vi "Vision Research Phantom Series PhCon PhGetVersion.vi"(0 "CN in":u32=1, 2 "VerSel":T1 items=["GV_CAMERA"=1, "GV_FIRMWARE"=2, "GV_FPGA"=3, "GV_PHCON"=4, "GV_CFA"=5, "GV_KERNEL"=6, "GV_MAGAZINE"=7], 5 "Error In (no error)":errorcluster) -> (14 "CN out":u32=1, 16 "pVersion":u32, 19 "Error Out":errorcluster)   [LabVIEW 2013, in "VRI.lvlib"]
doc: "PhCon.dll\n\nPhGetVersion\nHRESULT PhGetVersion(UINT CN, UINT VerSel UINT*pVersion);\n\nParameters Description\nCN (in) Camera number.\nVerSel (in) Code to select the wanted version.\npVersion (out) The version requested.\nReturn HRESULT (0=Ok)\nComments Get the versions of the camera hardware, firmware, dll, \n FPGAs or sensor CFA. Set the VerSel parameter to one \n of the below values:\n GV_CAMERA–get the camera hardware version\n GV_FIRMWARE-get the firmware version\n GV_FPGA-get the FPGAs version\n GV_PHCON-get the dll version\n GV_CFA-get the sensor CFA\n\n\nWritten by:\nBLOOMY CONTROLS, INC\nWINDSOR, CT 06095, USA\n860-298-9925\nwww.bloomy.com\nV1.0.0\nMay, 2004"
uses:
  VRI.lvlib
  _Type Defs/PhCon VerSel.ctl
  Phantom DLLs/PhCon.Dll
panel:
  # "For instructions on the use of this VI, press Ctrl+H to display the help window and move the mouse over the icon, controls, and indicators"
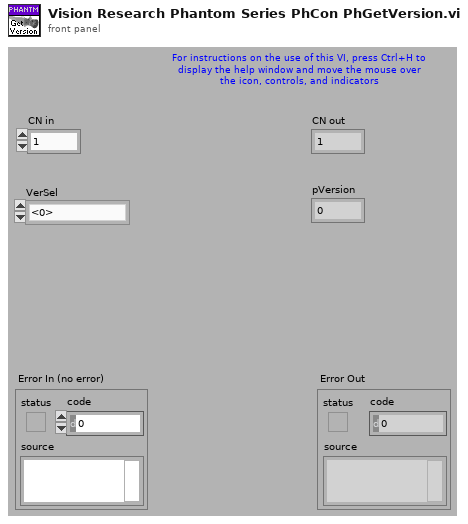
[diagram p1: front panel]
types:
  T1 = typedef "VRI.lvlib/PhCon VerSel.ctl" = u16
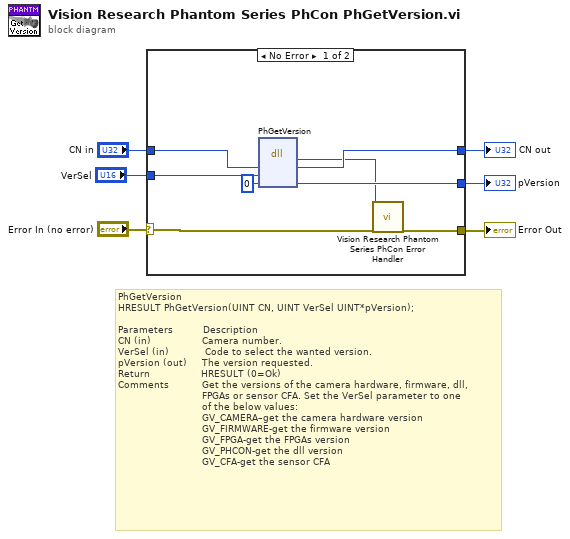
[diagram p0: block diagram]
diagram:
  # "PhGetVersion\nHRESULT PhGetVersion(UINT CN, UINT VerSel UINT*pVersion);\n\nParameters          Description\nCN (in)                 Camera number.\nVerSel (in)            Code to select the wanted version.\npVersion (out)     The version requested.\nReturn                 HRESULT (0=Ok)\nComments           Get the versions of the camera hardware, firmware, dll, \n                            FPGAs or sensor CFA. Set the VerSel parameter to one \n                            of the below values:\n                            GV_CAMERA–get the camera hardware version\n                            GV_FIRMWARE-get the firmware version\n                            GV_FPGA-get the FPGAs version\n                            GV_PHCON-get the dll version\n                            GV_CFA-get the sensor CFA"
  n1 = case shown="No Error" "Error In (no error)" {
    selector: "Error In (no error)" -> [w14 w16]
    tunnel: [w13 w16] -> w5
    tunnel: "CN in" -> [w12 w15]
    tunnel: [w11 w15] -> w3
    tunnel: "VerSel" -> [w10 _]
    tunnel: [w9 _] -> w1
    frame No Error {
      n2 = dll-call lib="C:/Projects/SDK/64-bit/Vision Research Phantom Series Labview Driver/Phantom DLLs/PhCon.dll" fn="PhGetVersion"("CN"=w12, "VerSel"=w10, "pVersion"=u32 0) -> ("HRESULT"=w8:i32, "CN"=w11:u32, "pVersion"=w9:u32)  [unwired: 3 in, 3 out]
      n3 = call "Vision Research Phantom Series PhCon Error Handler.vi"("ErrNo"=w8, "Error In (no error)"=w14) -> ("Error Out"=w13:errorcluster)  [unwired: 17 out]
    }
    frame Error {
    }
  }
  "Error Out" <- w5
  "CN out" <- w3
  "pVersion" <- w1
